vi "ElevatorSetpoints.vi"(8 "error in (no error)":errorcluster, 11 "ElevatorSetpoints":T1=enum."Rest") -> (0 "error out":errorcluster, 2 "OuterTargetHeight":dbl, 3 "Stage3TargetHeight":dbl)   [LabVIEW 2023]
doc: "NEEDS FINISHED-CURRENT HEIGHTS ARE GUESSES--Recieves a setpoint name and gives back a target position height (based on height of bottom of elevator) for the elevator. \nPositions are as follows:\nRest:\nL1:\nSource: \nL2:\nCoral1:\nL3:\nCoral2:\nL4:\n\nInputs:\n--ElevatorSetpoints--Enum\n\nOuputs:\n--TargetHeight--numeric--inches"
uses:
  ElevatorSetpointEnum.ctl
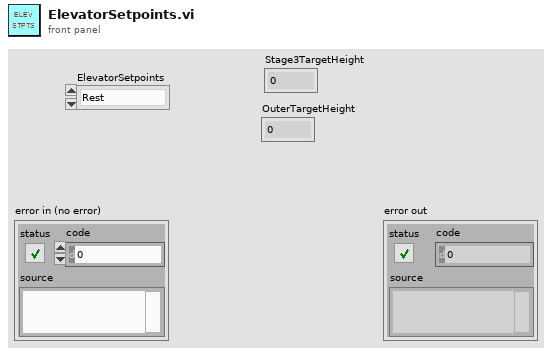
[diagram p1: front panel]
types:
  T1 = typedef "ElevatorSetpointEnum.ctl" = enum16{"Floor", "Rest", "Source", "L1", "L2", "Algae1", "L3", "Algae2", "L4", "Barge"}
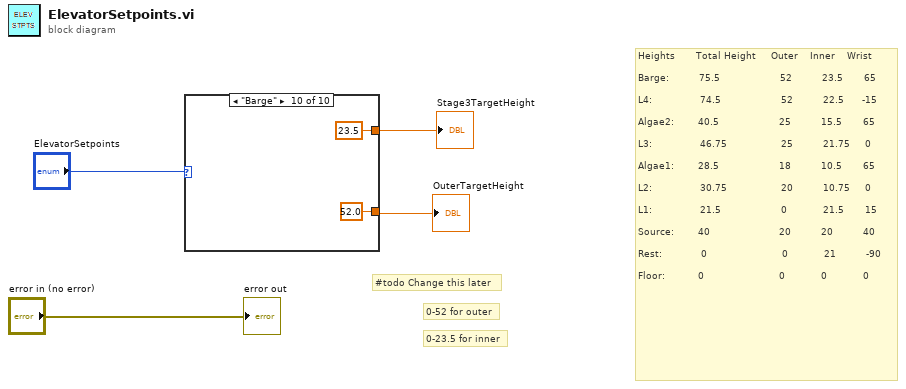
[diagram p0: block diagram]
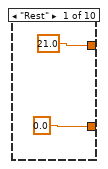
[diagram p2: hidden frame]
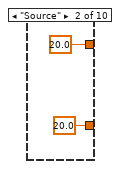
[diagram p3: hidden frame]
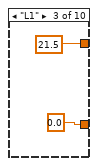
[diagram p4: hidden frame]
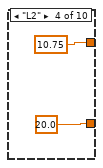
[diagram p5: hidden frame]
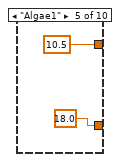
[diagram p6: hidden frame]
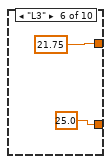
[diagram p7: hidden frame]
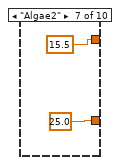
[diagram p8: hidden frame]
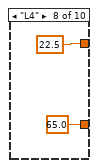
[diagram p9: hidden frame]
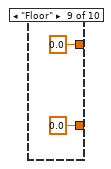
[diagram p10: hidden frame]
diagram:
  # "0-23.5 for inner"
  # "Heights       Total Height     Outer    Inner    Wrist\n\nBarge:          75.5                    52          23.5       65\n\nL4:                74.5                    52          22.5      -15\n\nAlgae2:        40.5                    25          15.5       65\n\nL3:                46.75                  25          21.75     0\n\nAlgae1:        28.5                    18          10.5       65\n\nL2:                30.75                  20          10.75     0\n\nL1:                21.5                    0            21.5       15\n\nSource:        40                       20          20          40\n\nRest:             0                         0            21          -90\n\nFloor:           0                         0            0            0"
  # "0-52 for outer"
  # "#todo Change this later"
  n1 = case shown="\"Barge\"" "ElevatorSetpoints" {
    tunnel: [0.0 ("TargetHeight") 20.0 ("TargetHeight") 0.0 ("TargetHeight") 20.0 ("TargetHeight") 18.0 ("TargetHeight") 25.0 ("TargetHeight") 25.0 ("TargetHeight") 65.0 ("TargetHeight") 0.0 ("TargetHeight") 52.0 ("TargetHeight")] -> w2
    tunnel: [21.0 ("TargetHeight") 20.0 ("TargetHeight") 21.5 ("TargetHeight") 10.75 ("TargetHeight") 10.5 ("TargetHeight") 21.75 ("TargetHeight") 15.5 ("TargetHeight") 22.5 ("TargetHeight") 0.0 ("TargetHeight") 23.5 ("TargetHeight")] -> w1
    frame "Rest" {
    }
    frame "Source" {
    }
    frame "L1" {
    }
    frame "L2" {
    }
    frame "Algae1" {
    }
    frame "L3" {
    }
    frame "Algae2" {
    }
    frame "L4" {
    }
    frame "Floor" {
    }
    frame "Barge" {
    }
  }
  "OuterTargetHeight" <- w2
  "Stage3TargetHeight" <- w1
  "error out" <- "error in (no error)"
